vi "retrieve token.vi"(8 "error in (no error)":errorcluster, 10 "Request URI in":string, 11 "Oauth2 in":refnum<class "Oauth2.lvclass">) -> (0 "error out":errorcluster, 2 "JSON Response":string, 3 "Oauth2 out":refnum<class "Oauth2.lvclass">)   [LabVIEW 2013, in "Oauth2.lvclass"]
uses:
  Oauth2.lvclass
  Oauth2.lvclass/Oauth2.ctl
  OauthClient/OAuthClient.lvclass
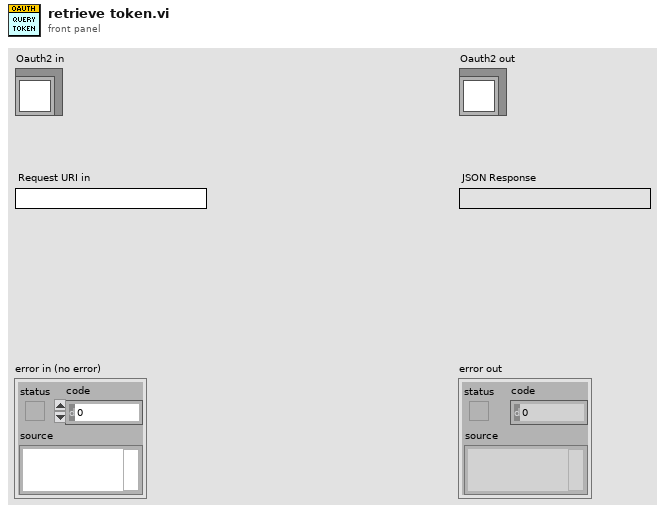
[diagram p1: front panel]
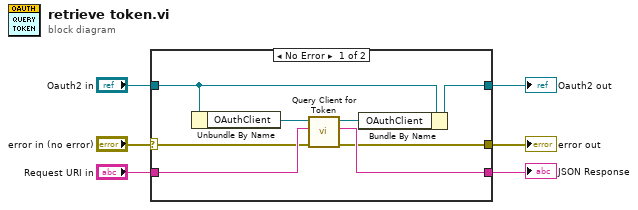
[diagram p0: block diagram]
diagram:
  n1 = case shown="No Error" "error in (no error)" {
    selector: "error in (no error)" -> [w8 w17]
    tunnel: [w7 w17] -> w5
    tunnel: [w13 w16] -> w3
    tunnel: "Oauth2 in" -> [w14 w16]
    tunnel: [w9 w15] -> w2
    tunnel: "Request URI in" -> [w10 w15]
    frame No Error {
      n2 = Unbundle By Name(w14) -> ("OAuthClient"=w12:refnum<class "OAuthClient.lvclass">)
      n3 = call-dynamic "Query Client for Token.vi"("error in (no error)"=w8, "Request URI"=w10, "OAuthClient in"=w12) -> ("error out"=w7:errorcluster, "Token Payload"=w9:string, "OAuthClient out"=w11:refnum<class "OAuthClient.lvclass">)  [unwired: 6 in]
      n4 = Bundle By Name(cluster=w14, "OAuthClient"=w11) -> (w13:refnum<class "Oauth2.lvclass">)
    }
    frame Error {
    }
  }
  "error out" <- w5
  "Oauth2 out" <- w3
  "JSON Response" <- w2
